vi "Chess.vi"(8 "column":i32, 9 "row":i32, 11 "State":enum16{"Initialize", "Play", "Read"}(ring)) -> (0 "Over?":bool, 1 "Message":string, 3 "Data":u16[][](array[numeric]))   [LabVIEW 2015]
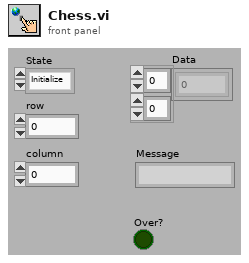
[diagram p1: front panel]
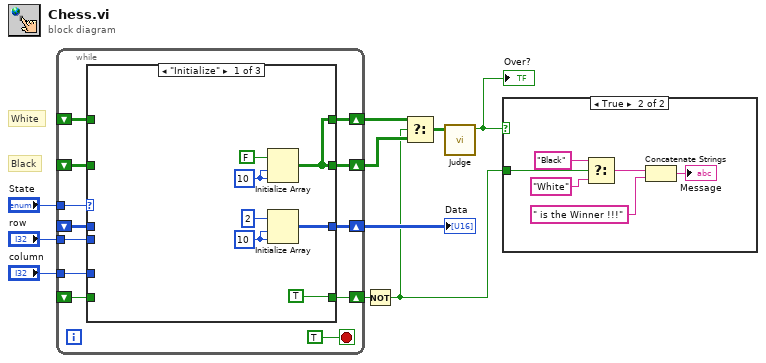
[diagram p0: block diagram]
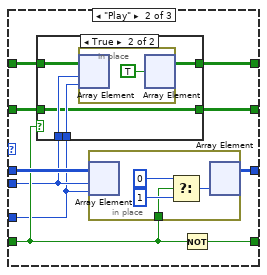
[diagram p3: hidden frame]
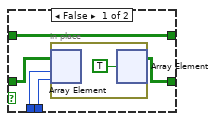
[diagram p4: hidden frame]
diagram:
  # "Black"
  # "White"
  n1 = while {
    tunnel: "State" -> [w22]
    shift-right: [w21] -> w7
    shift-left: _ -> [w20]
    shift-right: [w19] -> w6
    shift-left: _ -> [w18]
    tunnel: "row" -> [w17]
    tunnel: "column" -> [w16]
    shift-right: [w13] -> w5
    shift-left: _ -> [w15]
    shift-right: [w12] -> w4
    shift-left: _ -> [w14]
    stop <- TRUE stop-if-true
    n2 = case shown="\"Initialize\"" w22 {
      tunnel: [w27 w37 w59] -> w21
      tunnel: w20 -> [_ w38 w59]
      tunnel: [TRUE w39 w58] -> w19
      tunnel: w18 -> [_ w36 w58]
      tunnel: w17 -> [_ w32 _]
      tunnel: w16 -> [_ w31 _]
      tunnel: w15 -> [_ w35 w56]
      tunnel: w14 -> [_ w34 w57]
      tunnel: [w24 w30 w56] -> w13
      tunnel: [w24 w33 w57] -> w12
      frame "Initialize" {
        w26 = 10 ("dimension size")
        w28 = 10 ("dimension size")
        n3 = Initialize Array(FALSE, w26, w26) -> (w24:bool[][])
        n4 = Initialize Array(u16 2, w28, w28) -> (w27:u16[][])
      }
      frame "Play" {
        n5 = case shown="True" w36 {
          tunnel: w35 -> [w44 w46]
          tunnel: w34 -> [w40 w50]
          tunnel: [w40 w49] -> w33
          tunnel: w32 -> [w42 w48]
          tunnel: w31 -> [w41 w47]
          tunnel: [w43 w46] -> w30
          frame False {
            n6 = in-place {
              n7 = in-place-array #1(w44, w42, w41) -> ()  [unwired: 1 out]
              n8 = in-place-array #1(TRUE ("element")) -> (w43:bool[][])  [unwired: 2 out]
            }
          }
          frame True {
            n9 = in-place {
              n10 = in-place-array #2(w50, w48, w47) -> ()  [unwired: 1 out]
              n11 = in-place-array #2(TRUE ("element")) -> (w49:bool[][])  [unwired: 2 out]
            }
          }
        }
        n12 = in-place {
          in-place-border: w36 -> [w52]
          n13 = in-place-array #3(w38, w32, w31) -> ()  [unwired: 1 out]
          n14 = Select(t=u16 0 ("element"), s=w52, f=u16 1 ("element")) -> (s? t:f=w53:u16)
          n15 = in-place-array #3(w53) -> (w37:u16[][])  [unwired: 2 out]
        }
        n16 = Not(x=w36) -> (.not. x?=w39:bool)
      }
      frame "Read", Default {
      }
    }
  }
  "Data" <- w7
  n17 = Not(x=w6) -> (.not. x?=w2:bool)
  n18 = Select(t=w4, s=w2, f=w5) -> (s? t:f=w3:bool[][])
  n19 = call "Judge.vi"("chess"=w3) -> ("Over?"=w1:bool)  [unwired: 10 in]
  "Over?" <- w1
  n20 = case shown="True" w1 {
    tunnel: w2 -> [_ w61]
    frame False {
    }
    frame True {
      n21 = Select(t="Black" ("T button name (\"OK\")"), s=w61, f="White" ("T button name (\"OK\")")) -> (s? t:f=w64:string)
      n22 = Concatenate Strings(w64, " is the Winner !!!") -> (→"Message":string)
    }
  }
